vi "MainRT.vi"   [LabVIEW 2016]
uses:
  Controls/Message Structure.ctl
  Controls/Operational Modes.ctl
  Controls/Shutters.ctl
  Controls/Shutter Data.ctl
  Controls/Shutter States.ctl
  Controls/Shutter Message.ctl
  Controls/Flip Mirrors.ctl
  Controls/Mirror Data.ctl
  Controls/Flip Mirror Message.ctl
types:
  T1 = typedef "Message Structure.ctl" = cluster{"Data":variant, "Cmd":string}
  T2 = typedef "Shutter Message.ctl" = cluster{"Shutters":T3, "Op Mode":T6}
  T3 = typedef "Shutters.ctl" = cluster{"Science":T4, "LFCSim":T4, "ExtendFlat":T4, "SimFlat":T4, "Solar":T4}
  T4 = typedef "Shutter Data.ctl" = cluster{"Status":bool, "State":T5, "Time Stamps":cluster{"Open":timestamp, "Close":timestamp}, "Exposure Time":dbl}
  T5 = typedef "Shutter States.ctl" = enum16{"Open", "Close", "Wait", "Off", "Arm", "Idle"}
  T6 = typedef "Operational Modes.ctl" = enum16{"Sci", "Sci-LFC", "Solar", "Solar-LFC", "LFC", "LFC-Sim", "LFC-Both", "ThAr", "ThAr-LFC", "Flat", "ExtFlat", "ExtFlat-Sim", "ExtFlat-Both", "Qtz", "ExtQtz", "ExtQtz-Sim", "ExtQtz-Both", "Dark", "Manual", "Off"}
  T7 = typedef "Flip Mirror Message.ctl" = cluster{"Mirrors":T8, "Op Mode":T6}
  T8 = typedef "Flip Mirrors.ctl" = cluster{"ExtFlat":T9, "ThAr":T9, "Solar":T9}
  T9 = typedef "Mirror Data.ctl" = cluster{"Status":bool, "Time Stamp":timestamp}
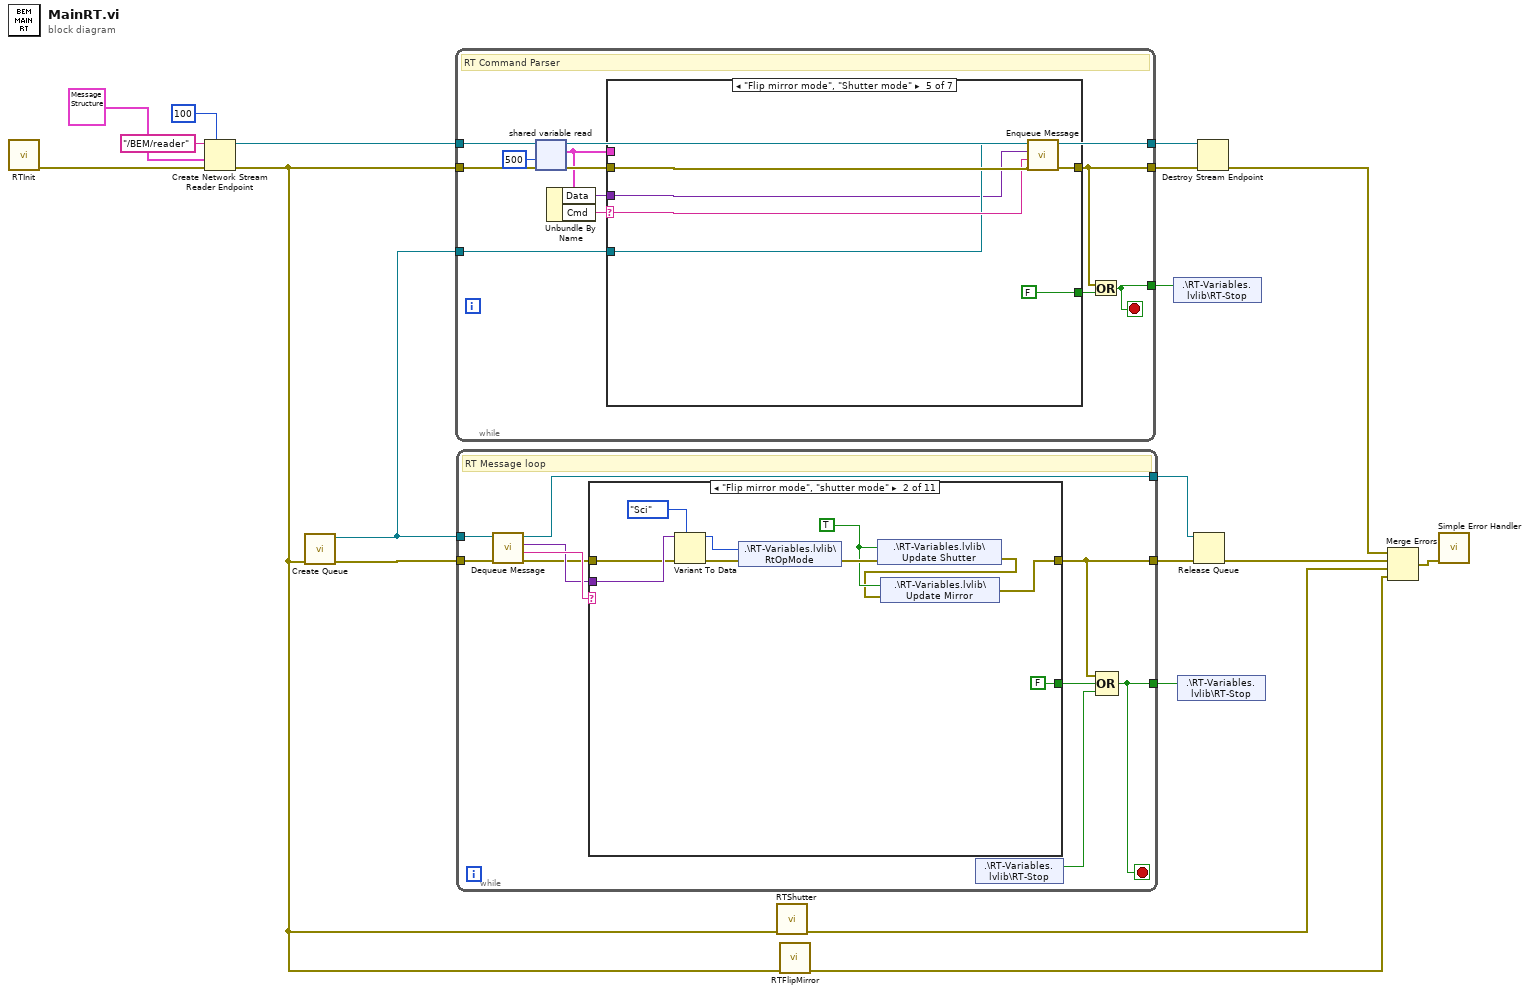
[diagram p0: block diagram]
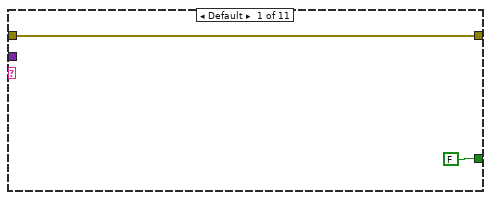
[diagram p2: hidden frame]
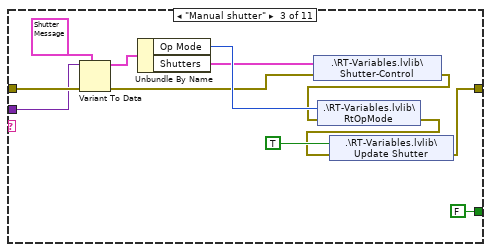
[diagram p3: hidden frame]
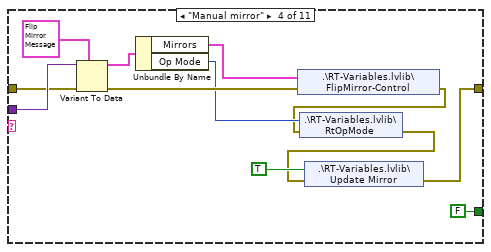
[diagram p4: hidden frame]
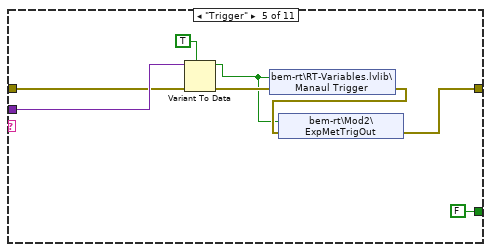
[diagram p5: hidden frame]
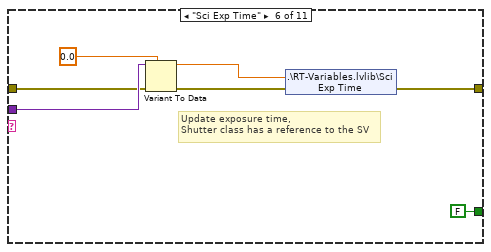
[diagram p6: hidden frame]
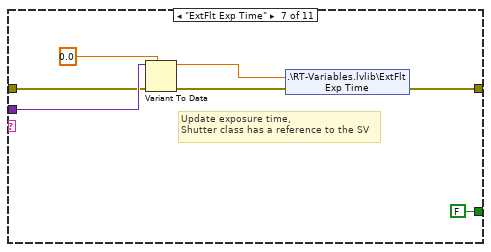
[diagram p7: hidden frame]
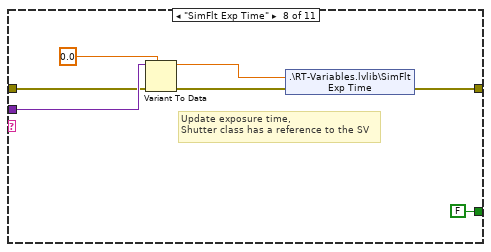
[diagram p8: hidden frame]
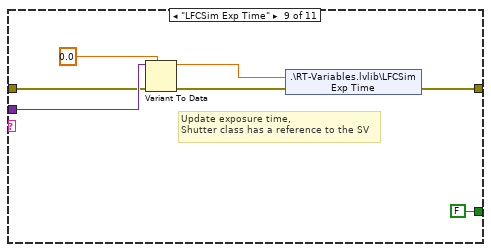
[diagram p9: hidden frame]
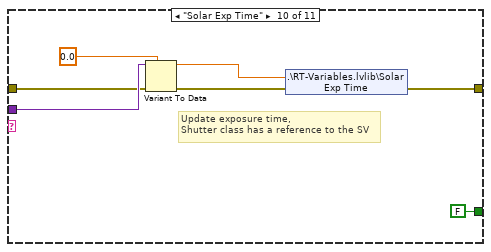
[diagram p10: hidden frame]
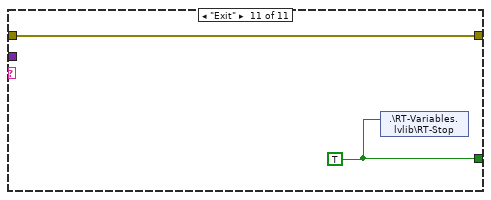
[diagram p11: hidden frame]
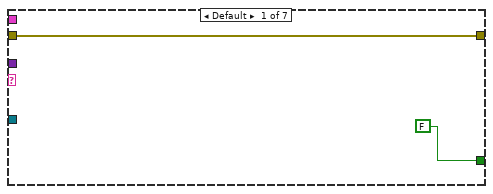
[diagram p12: hidden frame]
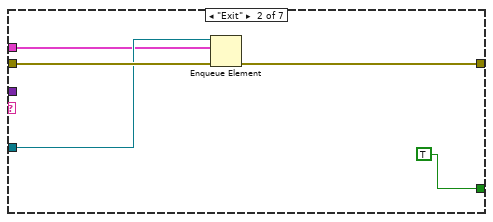
[diagram p13: hidden frame]
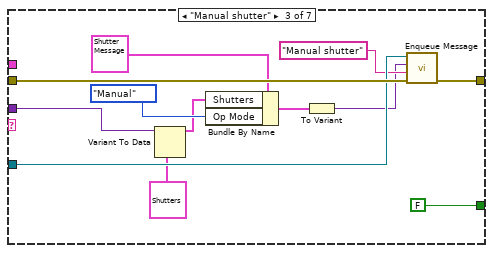
[diagram p14: hidden frame]
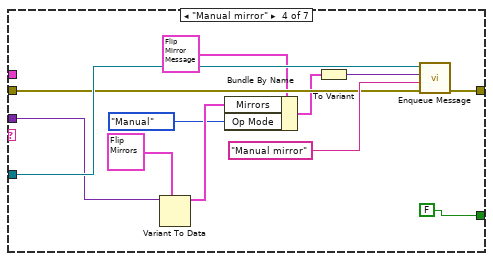
[diagram p15: hidden frame]
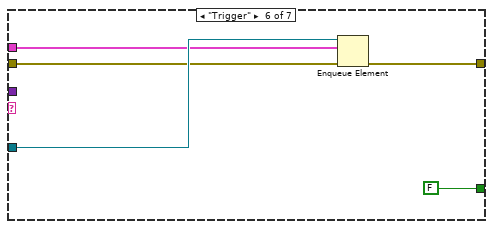
[diagram p16: hidden frame]
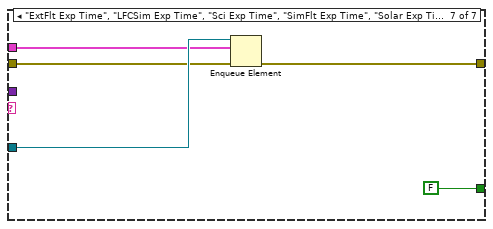
[diagram p17: hidden frame]
diagram:
  n1 = call "RTInit.vi"() -> ("error out"=w2:errorcluster)  [unwired: 11 in]
  n2 = Create Network Stream Reader Endpoint(7:100 ("reader buffer size"), 8:w2, 9:T1 {"Data"=variant, "Cmd"=""}, 11:"/BEM/reader" ("reader name")) -> (0:w1:errorcluster, 3:w17:refnum<k21>)  [unwired: 3 in]
  n3 = call "Create Queue.vi"("error in (no error)"=w1) -> ("error out"=w4:errorcluster, "Queue out"=w5:refnum<queue>)  [unwired: 9 in]
  n4 = while {
    tunnel: w1 -> [w31]
    tunnel: w17 -> [w30]
    tunnel: [w29] -> w15
    tunnel: [w24] -> w16
    tunnel: w5 -> [w23]
    tunnel: [w21] -> w11
    stop <- w21 stop-if-true
    # "RT Command Parser"
    n5 = shared-variable-read(w30, w31, 500 ("timeout ms (-1)")) -> (w29:refnum<k21>, w25:errorcluster, w22:T1)  [unwired: 1 out]
    n6 = Unbundle By Name(w22) -> ("Data"=w26:variant, "Cmd"=w28:string)
    n7 = case shown="\"Flip mirror mode\", \"Shutter mode\"" w28 {
      selector: w28 -> [_ _ _ _ w65 _ _]
      tunnel: [FALSE TRUE FALSE FALSE FALSE FALSE FALSE] -> w27
      tunnel: w26 -> [_ _ w49 w57 w63 _ _]
      tunnel: w25 -> [w32 w37 w45 w58 w66 w72 w77]
      tunnel: [w32 w36 w46 w59 w67 w71 w76] -> w24
      tunnel: w23 -> [_ w35 w44 w60 w64 w73 w78]
      tunnel: w22 -> [_ w34 _ _ _ w70 w75]
      frame Default {
      }
      frame "Exit" {
        n8 = Enqueue Element(queue=w35, element=w34, error in (no error)=w37) -> (error out=w36:errorcluster)  [unwired: 1 in, 2 out]
      }
      frame "Manual shutter" {
        n9 = Variant To Data(type=T3 {"Science"={"Status"=FALSE, "State"=enum."Open", "Time Stamps"={"Open"=timestamp(0 s since 1904-01-01), "Close"=timestamp(0 s since 1904-01-01)}, "Exposure Time"=0.0}, "LFCSim"={"Status"=FALSE, "State"=enum."Open", "Time Stamps"={"Open"=timestamp(0 s since 1904-01-01), "Close"=timestamp(0 s since 1904-01-01)}, "Exposure Time"=0.0}, "ExtendFlat"={"Status"=FALSE, "State"=enum."Open", "Time Stamps"={"Open"=timestamp(0 s since 1904-01-01), "Close"=timestamp(0 s since 1904-01-01)}, "Exposure Time"=0.0}, "SimFlat"={"Status"=FALSE, "State"=enum."Open", "Time Stamps"={"Open"=timestamp(0 s since 1904-01-01), "Close"=timestamp(0 s since 1904-01-01)}, "Exposure Time"=0.0}, "Solar"={"Status"=FALSE, "State"=enum."Open", "Time Stamps"={"Open"=timestamp(0 s since 1904-01-01), "Close"=timestamp(0 s since 1904-01-01)}, "Exposure Time"=0.0}} ("Shutters"), Variant=w49) -> (data=w39:T3)  [unwired: 1 in, 1 out]
        n10 = Bundle By Name(cluster=T2 {"Shutters"={"Science"={"Status"=FALSE, "State"=enum."Arm", "Time Stamps"={"Open"=timestamp(0 s since 1904-01-01), "Close"=timestamp(0 s since 1904-01-01)}, "Exposure Time"=0.0}, "LFCSim"={"Status"=FALSE, "State"=enum."Open", "Time Stamps"={"Open"=timestamp(0 s since 1904-01-01), "Close"=timestamp(0 s since 1904-01-01)}, "Exposure Time"=0.0}, "ExtendFlat"={"Status"=FALSE, "State"=enum."Open", "Time Stamps"={"Open"=timestamp(0 s since 1904-01-01), "Close"=timestamp(0 s since 1904-01-01)}, "Exposure Time"=0.0}, "SimFlat"={"Status"=FALSE, "State"=enum."Open", "Time Stamps"={"Open"=timestamp(0 s since 1904-01-01), "Close"=timestamp(0 s since 1904-01-01)}, "Exposure Time"=0.0}, "Solar"={"Status"=FALSE, "State"=enum."Open", "Time Stamps"={"Open"=timestamp(0 s since 1904-01-01), "Close"=timestamp(0 s since 1904-01-01)}, "Exposure Time"=0.0}}, "Op Mode"=enum."Sci"} ("Shutter Message"), "Shutters"=w39, "Op Mode"=Operational_Modes."Manual") -> (w47:T2)
        n11 = To Variant(anything=w47) -> (Variant=w42:variant)
        n12 = call "Enqueue Message.vi"("error in (no error)"=w45, "Cmd"="Manual shutter", "Data variant"=w42, "Queue In"=w44) -> ("error out"=w46:errorcluster)  [unwired: 7 in]
      }
      frame "Manual mirror" {
        n13 = Variant To Data(type=T8 {"ExtFlat"={"Status"=FALSE, "Time Stamp"=timestamp(0 s since 1904-01-01)}, "ThAr"={"Status"=FALSE, "Time Stamp"=timestamp(0 s since 1904-01-01)}, "Solar"={"Status"=FALSE, "Time Stamp"=timestamp(0 s since 1904-01-01)}} ("Mirrors"), Variant=w57) -> (data=w54:T8)  [unwired: 1 in, 1 out]
        n14 = Bundle By Name(cluster=T7 {"Mirrors"={"ExtFlat"={"Status"=FALSE, "Time Stamp"=timestamp(0 s since 1904-01-01)}, "ThAr"={"Status"=FALSE, "Time Stamp"=timestamp(0 s since 1904-01-01)}, "Solar"={"Status"=FALSE, "Time Stamp"=timestamp(0 s since 1904-01-01)}}, "Op Mode"=enum."Sci"} ("Flip Mirror Message"), "Mirrors"=w54, "Op Mode"=Operational_Modes."Manual") -> (w52:T7)
        n15 = To Variant(anything=w52) -> (Variant=w61:variant)
        n16 = call "Enqueue Message.vi"("error in (no error)"=w58, "Cmd"="Manual mirror", "Data variant"=w61, "Queue In"=w60) -> ("error out"=w59:errorcluster)  [unwired: 7 in]
      }
      frame "Flip mirror mode", "Shutter mode" {
        n17 = call "Enqueue Message.vi"("error in (no error)"=w66, "Cmd"=w65, "Data variant"=w63, "Queue In"=w64) -> ("error out"=w67:errorcluster)  [unwired: 7 in]
      }
      frame "Trigger" {
        n18 = Enqueue Element(queue=w73, element=w70, error in (no error)=w72) -> (error out=w71:errorcluster)  [unwired: 1 in, 2 out]
      }
      frame "ExtFlt Exp Time", "LFCSim Exp Time", "Sci Exp Time", "SimFlt Exp Time", "Solar Exp Time" {
        n19 = Enqueue Element(queue=w78, element=w75, error in (no error)=w77) -> (error out=w76:errorcluster)  [unwired: 1 in, 2 out]
      }
    }
    n20 = Or(x=w24, y=w27) -> (x .or. y?=w21:bool)
  }
  n21 = while {
    tunnel: w4 -> [w88]
    tunnel: w5 -> [w87]
    tunnel: [w83] -> w13
    tunnel: [w84] -> w12
    tunnel: [w80] -> w10
    stop <- w80 stop-if-true
    # "RT Message loop"
    n22 = call "Dequeue Message.vi"("error in (no error)"=w88, "Queue in"=w87) -> ("error out"=w79:errorcluster, "Cmd"=w86:string, "Data"=w85:variant, "Queue out"=w84:refnum<queue>)  [unwired: 6 in]
    n23 = case shown="\"Flip mirror mode\", \"shutter mode\"" w86 {
      tunnel: w85 -> [_ w93 w111 w122 w132 w139 w146 w153 w160 w167 _]
      tunnel: w79 -> [w89 w92 w112 w117 w131 w137 w144 w151 w158 w165 w169]
      tunnel: [FALSE FALSE FALSE FALSE FALSE FALSE FALSE FALSE FALSE FALSE w168] -> w82
      tunnel: [w89 w95 w104 w113 w126 w134 w141 w148 w155 w162 w169] -> w83
      frame Default {
      }
      frame "Flip mirror mode", "shutter mode" {
        w97 = TRUE ("Update?")
        n24 = Variant To Data(error in=w92, type=Operational_Modes."Sci" ("Operational Mode"), Variant=w93) -> (data=w94:T6, error out=w98:errorcluster)
        n25 = shared-variable ".\\RT-Variables.lvlib\\RtOpMode"(w94, error in=w98) -> (error out=w100:errorcluster)
        n26 = shared-variable ".\\RT-Variables.lvlib\\Update Shutter"(w97, error in=w100) -> (error out=w96:errorcluster)
        n27 = shared-variable ".\\RT-Variables.lvlib\\Update Mirror"(w97, error in=w96) -> (error out=w95:errorcluster)
      }
      frame "Manual shutter" {
        n28 = Variant To Data(error in=w112, type=T2 {"Shutters"={"Science"={"Status"=FALSE, "State"=enum."Arm", "Time Stamps"={"Open"=timestamp(0 s since 1904-01-01), "Close"=timestamp(0 s since 1904-01-01)}, "Exposure Time"=0.0}, "LFCSim"={"Status"=FALSE, "State"=enum."Open", "Time Stamps"={"Open"=timestamp(0 s since 1904-01-01), "Close"=timestamp(0 s since 1904-01-01)}, "Exposure Time"=0.0}, "ExtendFlat"={"Status"=FALSE, "State"=enum."Open", "Time Stamps"={"Open"=timestamp(0 s since 1904-01-01), "Close"=timestamp(0 s since 1904-01-01)}, "Exposure Time"=0.0}, "SimFlat"={"Status"=FALSE, "State"=enum."Open", "Time Stamps"={"Open"=timestamp(0 s since 1904-01-01), "Close"=timestamp(0 s since 1904-01-01)}, "Exposure Time"=0.0}, "Solar"={"Status"=FALSE, "State"=enum."Open", "Time Stamps"={"Open"=timestamp(0 s since 1904-01-01), "Close"=timestamp(0 s since 1904-01-01)}, "Exposure Time"=0.0}}, "Op Mode"=enum."Sci"} ("Shutter Message"), Variant=w111) -> (data=w107:T2, error out=w102:errorcluster)
        n29 = Unbundle By Name(w107) -> ("Op Mode"=w106:T6, "Shutters"=w101:T3)
        n30 = shared-variable ".\\RT-Variables.lvlib\\Shutter-Control"(w101, error in=w102) -> (error out=w103:errorcluster)
        n31 = shared-variable ".\\RT-Variables.lvlib\\RtOpMode"(w106, error in=w103) -> (error out=w105:errorcluster)
        n32 = shared-variable ".\\RT-Variables.lvlib\\Update Shutter"(TRUE ("Update?"), error in=w105) -> (error out=w104:errorcluster)
      }
      frame "Manual mirror" {
        n33 = Variant To Data(error in=w117, type=T7 {"Mirrors"={"ExtFlat"={"Status"=FALSE, "Time Stamp"=timestamp(0 s since 1904-01-01)}, "ThAr"={"Status"=FALSE, "Time Stamp"=timestamp(0 s since 1904-01-01)}, "Solar"={"Status"=FALSE, "Time Stamp"=timestamp(0 s since 1904-01-01)}}, "Op Mode"=enum."Sci"} ("Flip Mirror Message"), Variant=w122) -> (data=w120:T7, error out=w118:errorcluster)
        n34 = Unbundle By Name(w120) -> ("Mirrors"=w119:T8, "Op Mode"=w116:T6)
        n35 = shared-variable ".\\RT-Variables.lvlib\\FlipMirror-Control"(w119, error in=w118) -> (error out=w115:errorcluster)
        n36 = shared-variable ".\\RT-Variables.lvlib\\RtOpMode"(w116, error in=w115) -> (error out=w114:errorcluster)
        n37 = shared-variable ".\\RT-Variables.lvlib\\Update Mirror"(TRUE ("Update Mirror"), error in=w114) -> (error out=w113:errorcluster)
      }
      frame "Trigger" {
        n38 = Variant To Data(error in=w131, type=TRUE, Variant=w132) -> (data=w125:bool, error out=w129:errorcluster)
        n39 = shared-variable "bem-rt\\RT-Variables.lvlib\\Manaul Trigger"(w125, error in=w129) -> (error out=w127:errorcluster)
        n40 = shared-variable "bem-rt\\Mod2\\ExpMetTrigOut"(w125, error in=w127) -> (error out=w126:errorcluster)
      }
      frame "Sci Exp Time" {
        # "Update exposure time,\nShutter class has a reference to the SV"
        n41 = Variant To Data(error in=w137, type=0.0, Variant=w139) -> (data=w133:dbl, error out=w135:errorcluster)
        n42 = shared-variable ".\\RT-Variables.lvlib\\Sci Exp Time"(w133, error in=w135) -> (error out=w134:errorcluster)
      }
      frame "ExtFlt Exp Time" {
        # "Update exposure time,\nShutter class has a reference to the SV"
        n43 = Variant To Data(error in=w144, type=0.0, Variant=w146) -> (data=w140:dbl, error out=w142:errorcluster)
        n44 = shared-variable ".\\RT-Variables.lvlib\\ExtFlt Exp Time"(w140, error in=w142) -> (error out=w141:errorcluster)
      }
      frame "SimFlt Exp Time" {
        # "Update exposure time,\nShutter class has a reference to the SV"
        n45 = Variant To Data(error in=w151, type=0.0, Variant=w153) -> (data=w147:dbl, error out=w149:errorcluster)
        n46 = shared-variable ".\\RT-Variables.lvlib\\SimFlt Exp Time"(w147, error in=w149) -> (error out=w148:errorcluster)
      }
      frame "LFCSim Exp Time" {
        # "Update exposure time,\nShutter class has a reference to the SV"
        n47 = Variant To Data(error in=w158, type=0.0, Variant=w160) -> (data=w154:dbl, error out=w156:errorcluster)
        n48 = shared-variable ".\\RT-Variables.lvlib\\LFCSim Exp Time"(w154, error in=w156) -> (error out=w155:errorcluster)
      }
      frame "Solar Exp Time" {
        # "Update exposure time,\nShutter class has a reference to the SV"
        n49 = Variant To Data(error in=w165, type=0.0, Variant=w167) -> (data=w161:dbl, error out=w163:errorcluster)
        n50 = shared-variable ".\\RT-Variables.lvlib\\Solar Exp Time"(w161, error in=w163) -> (error out=w162:errorcluster)
      }
      frame "Exit" {
        w168 = TRUE
        n51 = shared-variable ".\\RT-Variables.lvlib\\RT-Stop"(w168) -> ()  [unwired: 1 in, 1 out]
      }
    }
    n52 = shared-variable ".\\RT-Variables.lvlib\\RT-Stop"() -> (w81:bool)  [unwired: 1 in, 1 out]
    n53 = Compound Arithmetic op=OR(w83, w82, w81) -> (w80:bool)
  }
  n54 = call "RTShutter.vi"("error in (no error)"=w1) -> ("error out"=w6:errorcluster)  [unwired: 10 in]
  n55 = call "RTFlipMirror.vi"("error in (no error)"=w1) -> ("error out"=w3:errorcluster)  [unwired: 10 in]
  n56 = shared-variable ".\\RT-Variables.lvlib\\RT-Stop"(w11) -> ()  [unwired: 1 in, 1 out]
  n57 = shared-variable ".\\RT-Variables.lvlib\\RT-Stop"(w10) -> ()  [unwired: 1 in, 1 out]
  n58 = Release Queue(queue=w12, error in (no error)=w13) -> (error out=w8:errorcluster)  [unwired: 1 in, 2 out]
  n59 = Destroy Stream Endpoint(8:w16, 11:w15) -> (0:w9:errorcluster)
  n60 = Merge Errors(w9, w8, w6, w3) -> (w7:errorcluster)
  n61 = call <vilib>:"Simple Error Handler.vi"("error in (no error)"=w7) -> ()  [unwired: 4 in, 5 out]
